vi "test_ccd_main.vi"(8 "error in (no error)":errorcluster) -> (0 "error out":errorcluster)   [LabVIEW 2023, in "horiba.test.lvlib"]
uses:
  horiba.test.lvlib
  Classes/CCD/CCD.lvclass
  C:/Projects/Horiba/horiba-labview-sdk/Source/Classes/GenericDevice/GenericDevice.lvclass
  <vilib>/addons/_JKI Toolkits/Caraya/classes/Test/Test.lvclass
  C:/Projects/Horiba/horiba-labview-sdk/Source/Classes/CCD/CCD.lvclass
panel:
  # "Connector Pane"
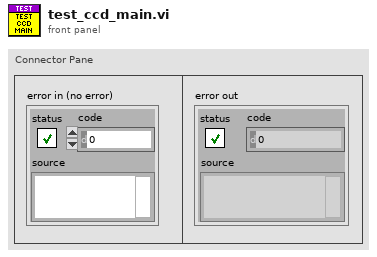
[diagram p1: front panel]
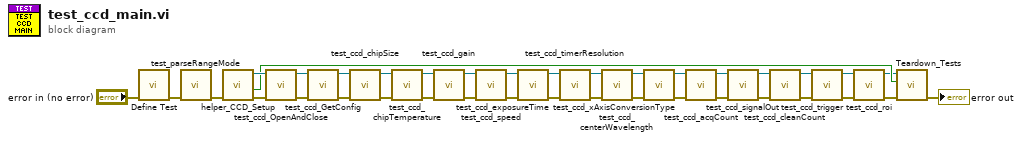
[diagram p0: block diagram]
diagram:
  n1 = call <vilib>:"Define Test.vi"("error in (no error)"="error in (no error)") -> ("error out"=w36:errorcluster)  [unwired: 9 in, 1 out]
  n2 = call "test_parseRangeMode.vi"("error in (no error)"=w36) -> ("error out"=w33:errorcluster)  [unwired: 10 in]
  n3 = call "helper_CCD_Setup.vi"("error in"=w33) -> ("error out"=w32:errorcluster, "Module Was Already Running?"=w30:bool, "CCD out"=w31:refnum<class "CCD.lvclass">)  [unwired: 7 in, 1 out]
  n4 = call "test_ccd_OpenAndClose.vi"("error in"=w32, "CCD in"=w31) -> ("error out"=w35:errorcluster, "CCD out"=w34:refnum<class "CCD.lvclass">)  [unwired: 8 in]
  n5 = call "test_ccd_GetConfig.vi"("error in"=w35, "CCD in"=w34) -> ("error out"=w28:errorcluster, "CCD out"=w29:refnum<class "CCD.lvclass">)  [unwired: 8 in]
  n6 = call "test_ccd_chipSize.vi"("error in"=w28, "CCD in"=w29) -> ("error out"=w26:errorcluster, "CCD out"=w27:refnum<class "CCD.lvclass">)  [unwired: 8 in]
  n7 = call "test_ccd_chipTemperature.vi"("error in"=w26, "CCD in"=w27) -> ("error out"=w24:errorcluster, "CCD out"=w23:refnum<class "CCD.lvclass">)  [unwired: 8 in]
  n8 = call "test_ccd_gain.vi"("error in"=w24, "CCD in"=w23) -> ("error out"=w21:errorcluster, "CCD out"=w22:refnum<class "CCD.lvclass">)  [unwired: 8 in]
  n9 = call "test_ccd_speed.vi"("error in"=w21, "CCD in"=w22) -> ("error out"=w20:errorcluster, "CCD out"=w19:refnum<class "CCD.lvclass">)  [unwired: 8 in]
  n10 = call "test_ccd_exposureTime.vi"("error in"=w20, "CCD in"=w19) -> ("error out"=w17:errorcluster, "CCD out"=w18:refnum<class "CCD.lvclass">)  [unwired: 8 in]
  n11 = call "test_ccd_timerResolution.vi"("error in"=w17, "CCD in"=w18) -> ("error out"=w15:errorcluster, "CCD out"=w16:refnum<class "CCD.lvclass">)  [unwired: 8 in]
  n12 = call "test_ccd_centerWavelength.vi"("error in"=w15, "CCD in"=w16) -> ("error out"=w13:errorcluster, "CCD out"=w14:refnum<class "CCD.lvclass">)  [unwired: 8 in]
  n13 = call "test_ccd_xAxisConversionType.vi"("error in"=w13, "CCD in"=w14) -> ("error out"=w12:errorcluster, "CCD out"=w10:refnum<class "CCD.lvclass">)  [unwired: 8 in]
  n14 = call "test_ccd_acqCount.vi"("error in"=w12, "CCD in"=w10) -> ("error out"=w11:errorcluster, "CCD out"=w8:refnum<class "CCD.lvclass">)  [unwired: 8 in]
  n15 = call "test_ccd_signalOut.vi"("error in"=w11, "CCD in"=w8) -> ("error out"=w9:errorcluster, "CCD out"=w6:refnum<class "CCD.lvclass">)  [unwired: 8 in]
  n16 = call "test_ccd_cleanCount.vi"("error in"=w9, "CCD in"=w6) -> ("error out"=w7:errorcluster, "CCD out"=w4:refnum<class "CCD.lvclass">)  [unwired: 8 in]
  n17 = call "test_ccd_trigger.vi"("error in"=w7, "CCD in"=w4) -> ("error out"=w5:errorcluster, "CCD out"=w2:refnum<class "CCD.lvclass">)  [unwired: 8 in]
  n18 = call "test_ccd_roi.vi"("error in"=w5, "CCD in"=w2) -> ("error out"=w3:errorcluster, "CCD out"=w1:refnum<class "CCD.lvclass">)  [unwired: 8 in]
  n19 = call "Teardown_Tests.vi"("error in"=w3, "Module Was Already Running?"=w30, "horiba.lvlib:GenericDevice"=w1) -> ("error out"=→"error out":errorcluster)  [unwired: 7 in, 1 out]
